vi "Go2XYZ (SubVI).vi"(0 ".NET Refnum in":refnum<k24>, 5 "Go to Coordinates":T2={"X [mm]"=25.0, "Y [mm]"=12.5, "Z [mm]"=5.0}, 7 "Axis Speeds":T4={"vX [mm/s]"=25.0, "vY [mm/s]"=12.5, "vZ [mm/s]"=5.0}, 11 "error in (no error)":errorcluster) -> (3 "completed":bool, 4 ".NET Refnum out":refnum<k24>, 6 "Final Position":T1, 14 "Initial Position":T3, 15 "error out":errorcluster)   [LabVIEW 2016]
uses:
  C:/Users/Aerotech/Documents/BNLStaveAssembly-blueprint/Bin/Aerotech.A3200.dll
  BNLStaveAssembly-blueprint/Bin/Aerotech.A3200.dll
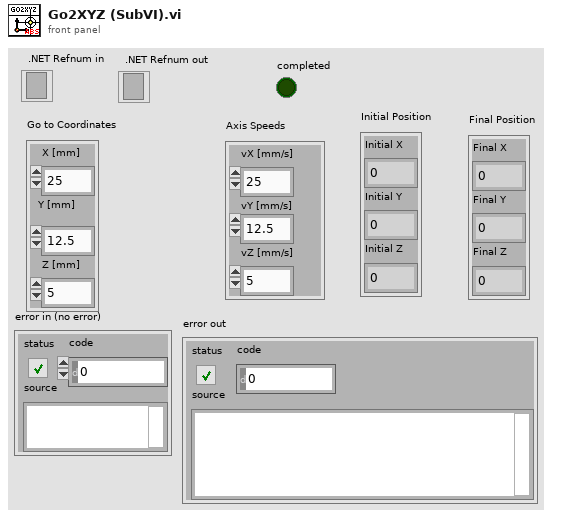
[diagram p1: front panel]
types:
  T1 = cluster{"Final X":dbl, "Final Y":dbl, "Final Z":dbl}
  T2 = cluster{"X [mm]":dbl, "Y [mm]":dbl, "Z [mm]":dbl}
  T3 = cluster{"Initial X":dbl, "Initial Y":dbl, "Initial Z":dbl}
  T4 = cluster{"vX [mm/s]":dbl, "vY [mm/s]":dbl, "vZ [mm/s]":dbl}
  T5 = cluster{"Go to X":dbl, "Go to Y":dbl, "Go to Z":dbl}
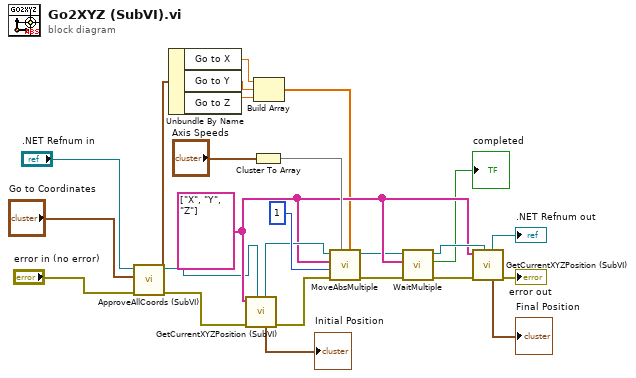
[diagram p0: block diagram]
diagram:
  w16 = string[] ["X", "Y", "Z"]
  n1 = call "ApproveAllCoords (SubVI).vi"("error in (no error)"="error in (no error)", "Go to Coordinates"="Go to Coordinates", "Controller .NET Refnum in"=".NET Refnum in") -> ("error out"=w14:errorcluster, "Approved Coordinates"=w9:T5, "Controller .NET Refnum out"=w10:refnum<k24>)  [unwired: 6 in]
  n2 = Unbundle By Name(w9) -> ("Go to X"=w11:dbl, "Go to Y"=w12:dbl, "Go to Z"=w13:dbl)
  n3 = call "GetCurrentXYZPosition (SubVI).vi"(".NET Refnum in - Device"=w10, "error in (no error)"=w14, "Axes Names"=w16) -> ("error out"=w24:errorcluster, "Current stage position"=→"Initial Position":T2, ".NET Refnum out  - Device"=w23:refnum<k24>)  [unwired: 3 in, 3 out]
  n4 = Cluster To Array(cluster="Axis Speeds") -> (array=w21:dbl[])
  n5 = Build Array(w11, w12, w13) -> (w6:dbl[])
  n6 = call "MoveAbsMultiple.vi"("positions"=w6, "speeds"=w21, "error in (no error)"=w24, "taskId"=1 ("taskNumber"), "axis names"=w16, "controller in"=w23) -> ("error out"=w5:errorcluster, "controller out"=w4:refnum<k24>)  [unwired: 4 in]
  n7 = call "WaitMultiple.vi"("error in (no error)"=w5, "axis names"=w16, "controller in"=w4) -> ("error out"=w18:errorcluster, "completed"=→"completed":bool, "controller out"=w20:refnum<k24>)  [unwired: 6 in]
  n8 = call "GetCurrentXYZPosition (SubVI).vi"(".NET Refnum in - Device"=w20, "error in (no error)"=w18, "Axes Names"=w16) -> ("error out"=→"error out":errorcluster, "Current stage position"=→"Final Position":T2, ".NET Refnum out  - Device"=→".NET Refnum out":refnum<k24>)  [unwired: 3 in, 3 out]
